vi "shell.vi"() -> ()   [LabVIEW 2021]
panel:
  in  "Path":path
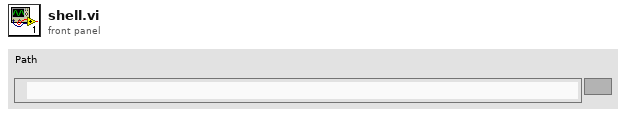
[diagram p1: front panel]
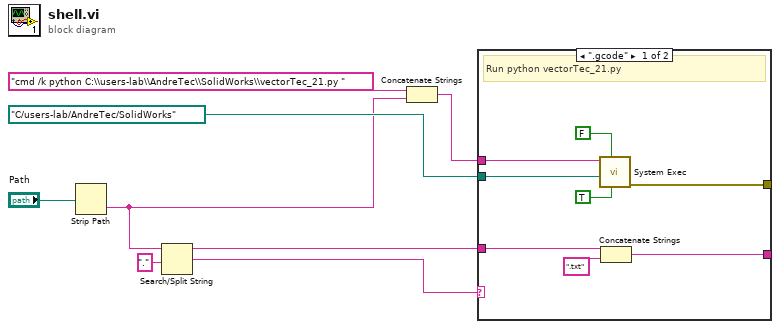
[diagram p0: block diagram]
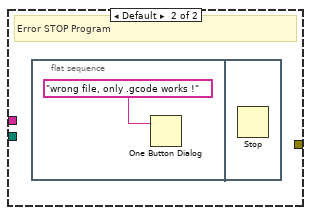
[diagram p2: hidden frame]
diagram:
  n1 = Strip Path(path="Path") -> (name=w2:string)  [unwired: 1 out]
  n2 = Search/Split String(string=w2, search string/char (-)=".") -> (substring before match=w1:string, match + rest of string=w3:string)  [unwired: 1 in, 1 out]
  n3 = Concatenate Strings("cmd /k python C:\\users-lab\\AndreTec\\SolidWorks\\vectorTec_21.py " ("command line"), w2) -> (w6:string)
  n4 = case shown="\".gcode\"" w3 {
    tunnel: path "C:/users-lab/AndreTec/SolidWorks" ("working directory") -> [w15 _]
    tunnel: w6 -> [w13 _]
    tunnel: [w12 _] -> _
    tunnel: w1 -> [w11 _]
    tunnel: [w9 _] -> _
    frame ".gcode" {
      # "Run python vectorTec_21.py"
      n5 = call <vilib>:"System Exec.vi"("run minimized? (F)"=TRUE, "wait until completion? (T)"=FALSE, "working directory"=w15, "command line"=w13) -> ("error out"=w12:errorcluster)  [unwired: 4 in, 3 out]
      n6 = Concatenate Strings(w11, ".txt" ("string")) -> (w9:string)
    }
    frame Default {
      # "Error STOP Program"
      n7 = flat-sequence {
        frame #0 {
          n8 = One Button Dialog(message="wrong file, only .gcode works !") -> ()  [unwired: 1 in, 1 out]
        }
        frame #1 {
          n9 = Stop() -> ()  [unwired: 1 in]
        }
      }
    }
  }
